vi "Write embedding_data.vi"(8 "error in (no error)":errorcluster, 10 "embedding_data":T1[](array[typedef]), 11 "message_vectors in":refnum<class "message_vectors.lvclass">) -> (0 "error out":errorcluster, 3 "message_vectors out":refnum<class "message_vectors.lvclass">)   [LabVIEW 2020, in "message_vectors.lvclass"]
uses:
  message_vectors.lvclass
  embedding.ctl
  message_vectors.lvclass/message_vectors.ctl
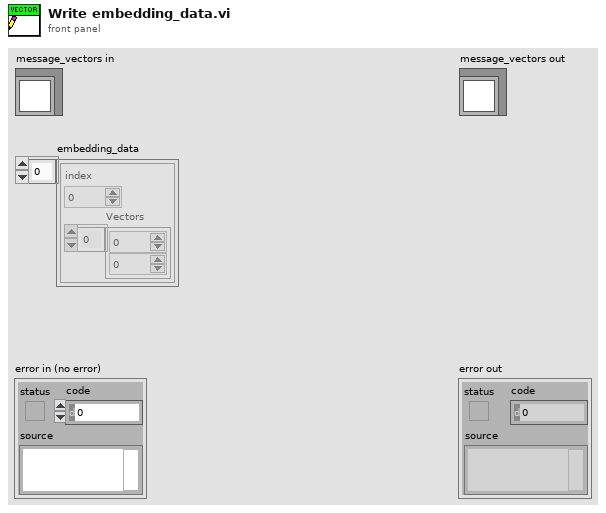
[diagram p1: front panel]
types:
  T1 = typedef "message_vectors.lvclass/embedding.ctl" = cluster{"index":u32, "Vectors":dbl[]}
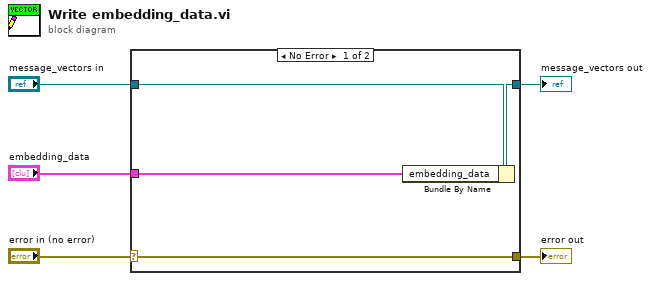
[diagram p0: block diagram]
diagram:
  n1 = case shown="No Error" "error in (no error)" {
    selector: "error in (no error)" -> [w9 w10]
    tunnel: [w9 w10] -> w4
    tunnel: [w7 w11] -> w2
    tunnel: "message_vectors in" -> [w8 w11]
    tunnel: "embedding_data" -> [w6 _]
    frame No Error {
      n2 = Bundle By Name(cluster=w8, "embedding_data"=w6) -> (w7:refnum<class "message_vectors.lvclass">)
    }
    frame Error {
    }
  }
  "error out" <- w4
  "message_vectors out" <- w2
